vi "Demo Workspace.vi"() -> ()   [LabVIEW 2017]
uses:
  <vilib>/httpClient/POSTBuffer.vi
  <vilib>/httpClient/LabVIEWHTTPClient.lvlib
  <vilib>/NI/VeriStand Web Service/vsws_api/vsws.lvlib
panel:
  in  "Autodetect":bool
  out "Echoed":string
  in  "To Echo":string
  out "Random Number":dbl
  in  "Echo":bool
  in  "Random":bool
  in  "queue":string
  in  "Stop Button":bool
  in  "GetVersion":bool
  out "version":string
  out "cmd":string
  out "response":string
  in  "ip":string
  in  "port":i32=8002
  out "url":string
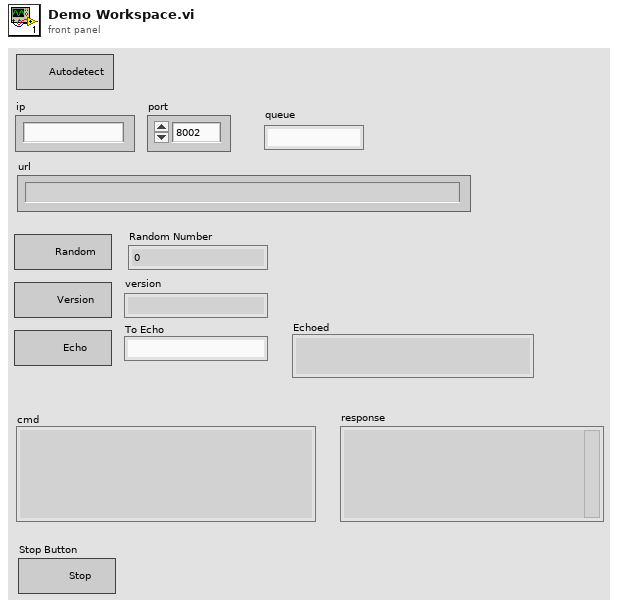
[diagram p1: front panel]
types:
  T1 = typedef "LabVIEWHTTPClient.lvlib/ClientHandle.ctl" = refnum<k1>
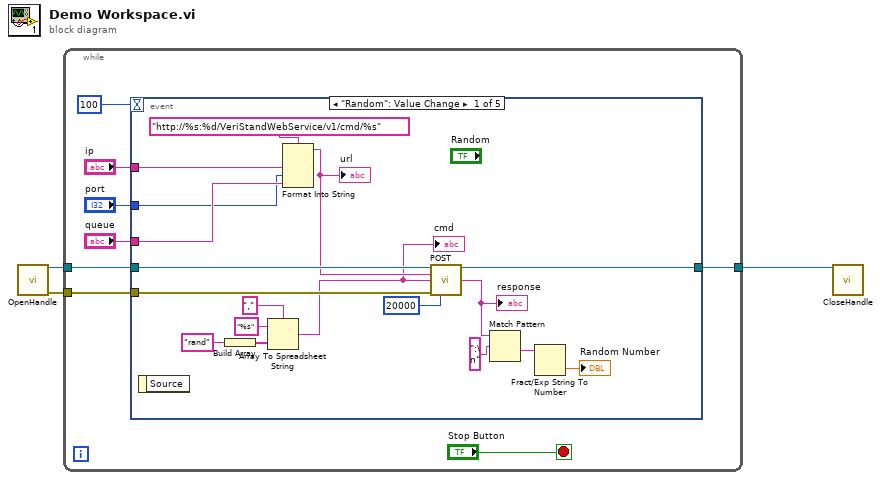
[diagram p0: block diagram]
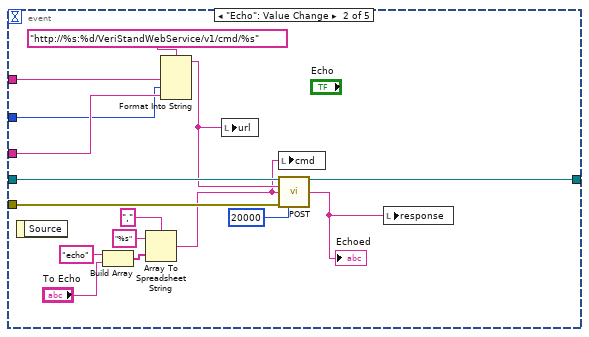
[diagram p2: hidden frame]
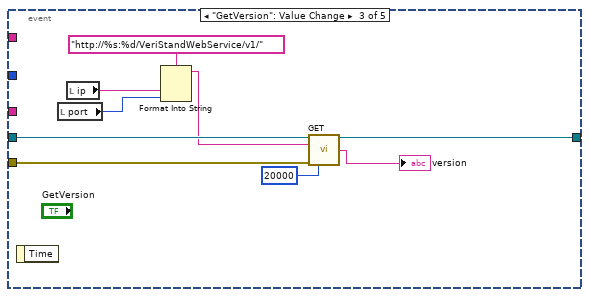
[diagram p3: hidden frame]
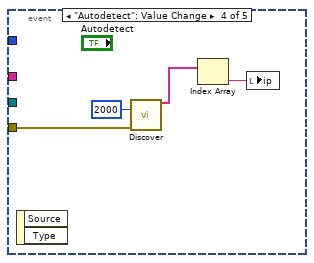
[diagram p4: hidden frame]
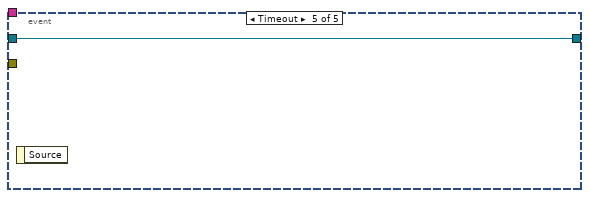
[diagram p5: hidden frame]
diagram:
  n1 = call <vilib>:"OpenHandle.vi"() -> ("client handle out"=w3:T1, "error out"=w2:errorcluster)  [unwired: 14 in]
  n2 = while {
    tunnel: w3 -> [w11]
    tunnel: w2 -> [w10]
    tunnel: [w9] -> w1
    stop <- "Stop Button" stop-if-true
    n3 = event shown="[0] \"Random\": Value Change" {
      selector: _ -> [_ _ _ _ _]
      dyn-events: _ -> [_ _ _ _ _]
      timeout: 100 -> [_ _ _ _ _]
      tunnel: w11 -> [w29 w45 w54 _ w59]
      tunnel: w10 -> [w28 w44 w53 w58 _]
      tunnel: [w27 w43 w52 _ w59] -> w9
      tunnel: "queue" -> [w19 w36 _ _ _]
      tunnel: "port" -> [w18 w35 _ _ _]
      tunnel: "ip" -> [w17 w34 _ _ _]
      event "Random": Value Change {
        n4 = event-data() -> ()  [unwired: 1 in, 1 out]
        n5 = Build Array("rand") -> (w22:string[])
        n6 = Array To Spreadsheet String(delimiter (Tab)=",", array=w22, 3:"%s" ("format string")) -> (spreadsheet string=w15:string)
        "cmd" <- w15
        n7 = Format Into String(format string="http://%s:%d/VeriStandWebService/v1/cmd/%s" ("url"), w17, w18, w19) -> (resulting string=w24:string)  [unwired: 2 in, 1 out]
        "url" <- w24
        n8 = call-poly <vilib>:"POST.vi"("client handle"=w29, "url"=w24, "buffer"=w15, "error in (no error)"=w28, "timeout (10000)"=20000) -> ("client handle out"=w27:T1, "body"=w14:string)  [unwired: 7 in, 2 out]
        "response" <- w14
        n9 = Match Pattern(string=w14, regular expression=":\n") -> (after substring=w12:string)  [unwired: 1 in, 3 out]
        n10 = Fract/Exp String To Number(string=w12) -> (number=→"Random Number":dbl)  [unwired: 3 in, 1 out]
      }
      event "Echo": Value Change {
        n11 = event-data() -> ()  [unwired: 1 in, 1 out]
        n12 = Build Array("echo", "To Echo") -> (w39:string[])
        n13 = Array To Spreadsheet String(delimiter (Tab)=",", array=w39, 3:"%s" ("format string")) -> (spreadsheet string=w30:string)
        n14 = Format Into String(format string="http://%s:%d/VeriStandWebService/v1/cmd/%s" ("url"), w34, w35, w36) -> (resulting string=w33:string)  [unwired: 2 in, 1 out]
        n15 = local write "url"(w33) -> ()
        n16 = local write "cmd"(w30) -> ()
        n17 = call-poly <vilib>:"POST.vi"("client handle"=w45, "url"=w33, "buffer"=w30, "error in (no error)"=w44, "timeout (10000)"=20000) -> ("client handle out"=w43:T1, "body"=w31:string)  [unwired: 7 in, 2 out]
        "Echoed" <- w31
        n18 = local write "response"(w31) -> ()
      }
      event "GetVersion": Value Change {
        n19 = event-data() -> ()  [unwired: 1 in, 1 out]
        n20 = local read "port"() -> (w48:i32)
        n21 = local read "ip"() -> (w49:string)
        n22 = Format Into String(format string="http://%s:%d/VeriStandWebService/v1/" ("url"), w49, w48) -> (resulting string=w46:string)  [unwired: 2 in, 1 out]
        n23 = call <vilib>:"GET.vi"("client handle"=w54, "url"=w46, "error in (no error)"=w53, "timeout (10000)"=20000) -> ("client handle out"=w52:T1, "body"=→"version":string)  [unwired: 8 in, 2 out]
      }
      event "Autodetect": Value Change {
        n24 = event-data() -> ()  [unwired: 1 in, 2 out]
        n25 = call <vilib>:"Discover.vi"("discovery time (ms)"=u16 2000, "error in (no error)"=w58) -> ("Discovered"=w56:string[])  [unwired: 12 in, 1 out]
        n26 = Index Array(array=w56) -> (element=w55:string)  [unwired: 1 in]
        n27 = local write "ip"(w55) -> ()
      }
      event Timeout {
        n28 = event-data() -> ()  [unwired: 1 in, 1 out]
      }
    }
  }
  n29 = call <vilib>:"CloseHandle.vi"("client handle"=w1) -> ()  [unwired: 14 in, 1 out]
